vi "FPGA_PPG_start.vi"(0 "resource_in":refnum<visa-resource-name>, 2 "start_addr":u32, 5 "error in (no error)":errorcluster) -> (14 "resource_out":refnum<visa-resource-name>, 19 "error out":errorcluster)   [LabVIEW 2014, in "NI-FPGA_PPG_Driver.lvlib"]
doc: "Starts the FPGA target with specified command address.\n\nContact: Falk Ziegler, eMail: ziegler@physik.uni-greifswald.de"
uses:
  NI-FPGA_PPG_Driver.lvlib
  FPGA_PPG_error_type.ctl
  FPGA_PPG_action_type.ctl
  <vilib>/rvi/errors/niLvFpgaAdjustHostInterfaceError.vi
  <vilib>/rvi/interface/nirviReadWriteControl/nirviReadWriteControl.xnode
  FPGA_PPG_vi_ref.ctl
  target/FPGA_target_state_type.ctl
  FPGA Bitfiles/TiTaProj_COF_PPG_80MHz.lvbitx
  NiFpgaLv.dll
panel:
  in  "errorCodes":T1
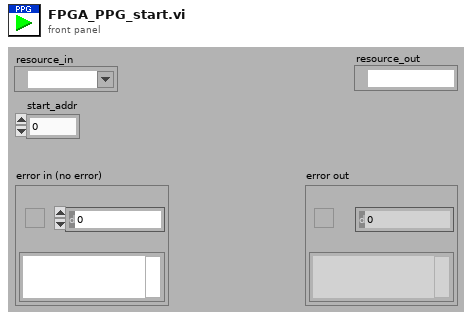
[diagram p1: front panel]
types:
  T1 = typedef "NI-FPGA_PPG_Driver.lvlib/FPGA_PPG_error_type.ctl" = enum16{"no error", "resource not initialized (no commands and invalid mem address)", "wrong memory address (address > Nof commands)", "invalid time value (probably too short)", "cannot start FPGA because one or more errors occured", "FIFO (internal) empty unexpectedly", "DMA FIFO (download from host) full unexpectedly", "checking number of commands: failed", "unknown error 8", "unknown error 9", "unknown error 10", "unknown error 11", "unknown error 12", "unknown error 13", "unknown error 14", "unknown error 15", "unknown error 16", "unknown error 17", "unknown error 18", "unknown error 19", "can't change state while pattern output is in progress"}
  T2 = typedef "NI-FPGA_PPG_Driver.lvlib/FPGA_PPG_action_type.ctl" = enum16{"GET", "SET", "REMOVE"}
  T3 = typedef "NI-FPGA_PPG_Driver.lvlib/FPGA_PPG_vi_ref.ctl" = refnum<k20>
  T4 = typedef "NI-FPGA_PPG_Driver.lvlib/FPGA_target_state_type.ctl" = enum16{"idle", "reset", "query", "load", "run", "stopped"}
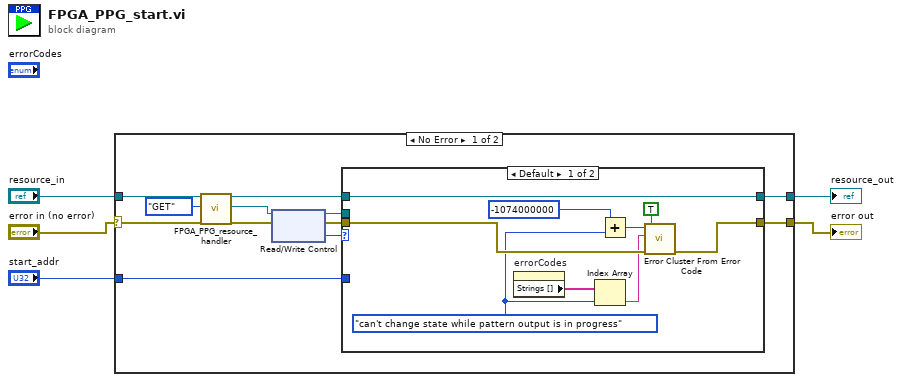
[diagram p0: block diagram]
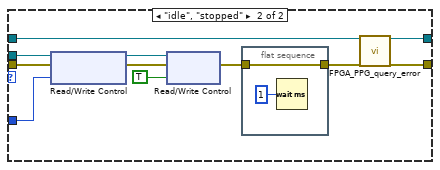
[diagram p2: hidden frame]
diagram:
  n1 = case shown="No Error" "error in (no error)" {
    selector: "error in (no error)" -> [w16 w41]
    tunnel: [w9 w41] -> w4
    tunnel: "start_addr" -> [w11 _]
    tunnel: "resource_in" -> [w17 w40]
    tunnel: [w8 w40] -> w1
    frame No Error {
      n2 = call "FPGA_PPG_resource_handler.vi"("resource_in"=w17, "action"=FPGA_PPG_action_type."GET", "error in (no error)"=w16) -> ("resource_out"=w14:refnum<visa-resource-name>, "FPGA VI Reference Out"=w7:T3, "error out"=w15:errorcluster)  [unwired: 14 in]
      n3 = xnode "Read/Write Control"("FPGA VI Reference In"=w7, "error in"=w15) -> ("FPGA VI Reference Out"=w12:T3, "error out"=w13:errorcluster, "state"=w10:T4)
      n4 = case shown="Default" w10 {
        tunnel: w14 -> [w26 w30]
        tunnel: w13 -> [w25 w36]
        tunnel: w12 -> [_ w37]
        tunnel: w11 -> [_ w35]
        tunnel: [w26 w29] -> w8
        tunnel: [w24 w27] -> w9
        frame Default {
          w18 = FPGA_PPG_error_type."can't change state while pattern output is in progress" ("errorCodes")
          n5 = property on="errorCodes" class="Enum (strict)"() -> ("Strings []"=w22:string[])  [unwired: 2 in, 2 out]
          n6 = Index Array(array=w22, index=w18) -> (element=w21:string)
          n7 = Add(x=-1074000000 ("error code (0)"), y=w18) -> (x+y=w19:i32)
          n8 = call <vilib>:"Error Cluster From Error Code.vi"("show call chain? (False)"=TRUE, "error in (no error)"=w25, "error message (\"\")"=w21, "error code (0)"=w19) -> ("error out"=w24:errorcluster)  [unwired: 5 in]
        }
        frame "idle", "stopped" {
          n9 = xnode "Read/Write Control"("FPGA VI Reference In"=w37, "error in"=w36, "mem_addr"=w35) -> ("FPGA VI Reference Out"=w34:T3, "error out"=w33:errorcluster)
          n10 = xnode "Read/Write Control"("FPGA VI Reference In"=w34, "error in"=w33, "run"=TRUE) -> ("error out"=w31:errorcluster)  [unwired: 1 out]
          n11 = flat-sequence {
            tunnel: w31 -> [w38]
            tunnel: [w38] -> w28
            frame #0 {
              n12 = Wait (ms)(milliseconds to wait=u32 1) -> ()  [unwired: 1 out]
            }
          }
          n13 = call "FPGA_PPG_query_error.vi"("resource_in"=w30, "error in (no error)"=w28) -> ("resource_out"=w29:refnum<visa-resource-name>, "error out"=w27:errorcluster)  [unwired: 16 in]
        }
      }
    }
    frame Error {
    }
  }
  "error out" <- w4
  "resource_out" <- w1
